vi "Expand Specified Item.vi"(8 "error in (no error)":errorcluster, 10 "Tag":string, 11 "TreeControl in":refnum<vi>) -> (0 "error IO":errorcluster, 3 "TreeControl in 2":refnum<vi>)   [LabVIEW 2021]
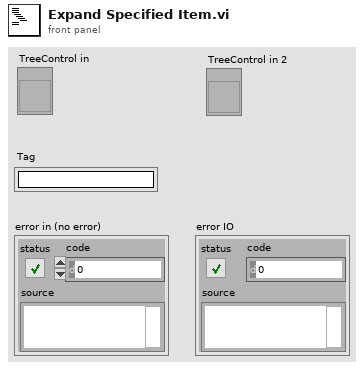
[diagram p1: front panel]
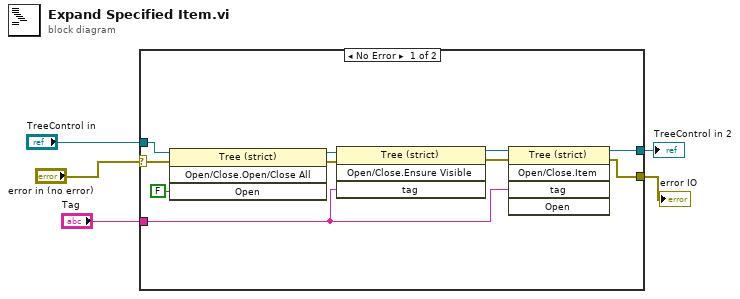
[diagram p0: block diagram]
diagram:
  n1 = case shown="No Error" "error in (no error)" {
    selector: "error in (no error)" -> [w12 w16]
    tunnel: "TreeControl in" -> [w13 w17]
    tunnel: "Tag" -> [w6 _]
    tunnel: [w8 w17] -> w1
    tunnel: [w7 w16] -> w2
    frame No Error {
      n2 = invoke class="Tree (strict)" method="Open/Close.Open/Close All"(reference=w13, error in=w12, "Open"=FALSE ("Open?")) -> (reference out=w14:refnum<vi>, error out=w15:errorcluster)  [unwired: 1 in, 2 out]
      n3 = invoke class="Tree (strict)" method="Open/Close.Ensure Visible"(reference=w14, error in=w15, "tag"=w6) -> (reference out=w10:refnum<vi>, error out=w9:errorcluster)  [unwired: 1 in, 2 out]
      n4 = invoke class="Tree (strict)" method="Open/Close.Item"(reference=w10, error in=w9, "tag"=w6) -> (reference out=w8:refnum<vi>, error out=w7:errorcluster)  [unwired: 2 in, 3 out]
    }
    frame Error {
    }
  }
  "error IO" <- w2
  "TreeControl in 2" <- w1
